vi "Read Recipe.vi"(8 "error in (no error)":errorcluster, 11 "MASTER in":refnum<class "MASTER.lvclass">) -> (0 "error out":errorcluster, 3 "MASTER out":refnum<class "MASTER.lvclass">)   [LabVIEW 2014, in "Files Library.lvlib" / "MASTER.lvclass"]
uses:
  MASTER/MASTER.lvclass
  CONTROL/RecipeIndicatorTypeDef.ctl
  CONTROL/Recipes Indicators.ctl
  MASTER/MASTER.lvclass/MASTER.ctl
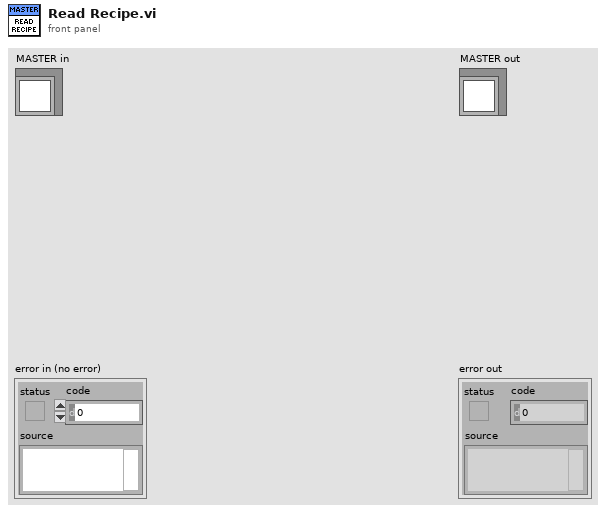
[diagram p1: front panel]
types:
  T1 = typedef "RecipeIndicatorTypeDef.ctl" = T2[]
  T2 = typedef "Recipes Indicators.ctl" = cluster{"Speed":string, "Temperature SP":string, "Time Limit":string, "Direction":string}
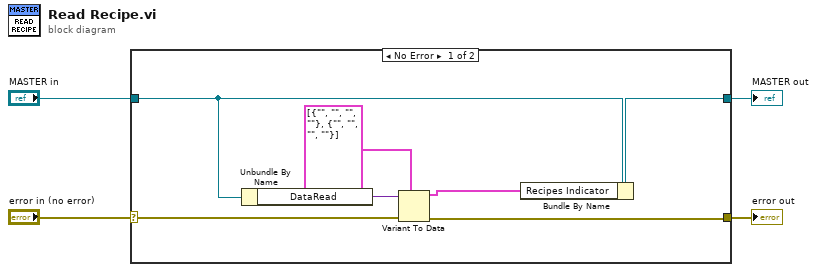
[diagram p0: block diagram]
diagram:
  n1 = case shown="No Error" "error in (no error)" {
    selector: "error in (no error)" -> [w9 w13]
    tunnel: [w8 w13] -> w3
    tunnel: [w10 w12] -> w1
    tunnel: "MASTER in" -> [w7 w12]
    frame No Error {
      n2 = Unbundle By Name(w7) -> ("DataRead"=w11:variant)
      n3 = Variant To Data(error in=w9, type=T1 [{"Speed"="", "Temperature SP"="", "Time Limit"="", "Direction"=""}, {"Speed"="", "Temperature SP"="", "Time Limit"="", "Direction"=""}] ("Recipes Indicator"), Variant=w11) -> (data=w6:T1, error out=w8:errorcluster)
      n4 = Bundle By Name(cluster=w7, "Recipes Indicator"=w6) -> (w10:refnum<class "MASTER.lvclass">)
    }
    frame Error {
    }
  }
  "error out" <- w3
  "MASTER out" <- w1
